vi "VariableGet.vi"(8 "error in (no error)":errorcluster, 10 "VariableName":string, 11 "VariableManager in":refnum<class "VariableManager.lvclass">) -> (0 "error out":errorcluster, 2 "Variable":refnum<class "Variable.lvclass">, 3 "VariableManager out":refnum<class "VariableManager.lvclass">)   [LabVIEW 2013, in "VariableManager.lvclass"]
doc: "Return variable definition of VariableName.\n\nAn error is thrown if a VariableName does not exist."
uses:
  VariableManager.lvclass
  Variable/Variable.lvclass
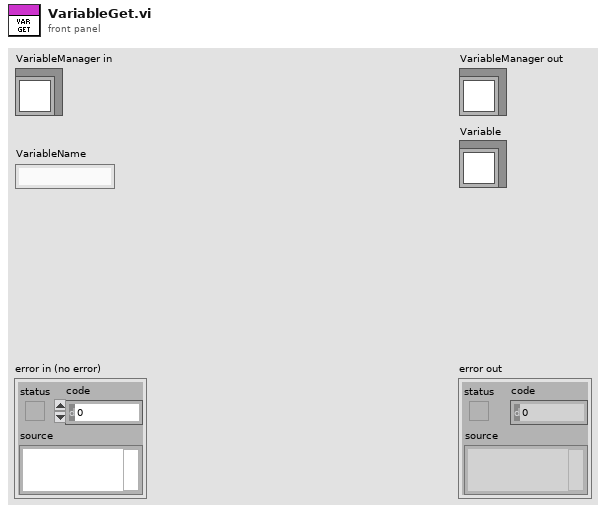
[diagram p1: front panel]
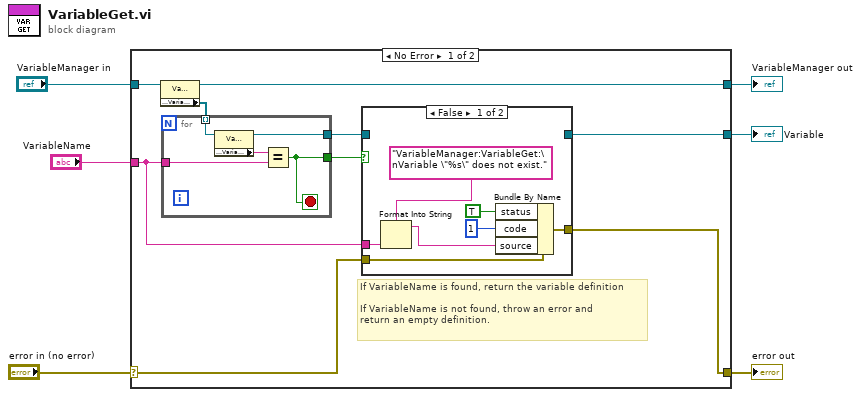
[diagram p0: block diagram]
diagram:
  n1 = case shown="No Error" "error in (no error)" {
    selector: "error in (no error)" -> [w9 w31]
    tunnel: [w8 w31] -> w5
    tunnel: [w14 w30] -> w3
    tunnel: "VariableManager in" -> [w15 w30]
    tunnel: "VariableName" -> [w7 _]
    tunnel: [w11 _] -> w1
    frame No Error {
      # "If VariableName is found, return the variable definition\n\nIf VariableName is not found, throw an error and\nreturn an empty definition."
      n2 = property class="VariableManager.lvclass"(reference=w15) -> (reference out=w14:refnum<class "VariableManager.lvclass">, "Accessors:Variables"=w13:refnum<class "Variable.lvclass">[])  [unwired: 1 in, 1 out]
      n3 = for {
        tunnel: w13 -> [w29] mode=indexing
        tunnel: w7 -> [w27]
        tunnel: [w26] -> w10
        tunnel: [w25] -> w12
        stop <- w26 stop-if-true
        n4 = property class="Variable.lvclass"(reference=w29) -> (reference out=w25:refnum<class "Variable.lvclass">, "Accessors:VariableName"=w28:string)  [unwired: 1 in, 1 out]
        n5 = Equal?(x=w28, y=w27) -> (x = y?=w26:bool)
      }
      n6 = case shown="False" w10 {
        tunnel: w12 -> [_ w23]
        tunnel: [_ w23] -> w11
        tunnel: w9 -> [w22 w24]
        tunnel: w7 -> [w18 _]
        tunnel: [w16 w24] -> w8
        frame False {
          n7 = Format Into String(format string="VariableManager:VariableGet:\nVariable \"%s\" does not exist.", w18) -> (resulting string=w17:string)  [unwired: 2 in, 1 out]
          n8 = Bundle By Name(cluster=w22, "status"=TRUE, "code"=1, "source"=w17) -> (w16:errorcluster)
        }
        frame True {
        }
      }
    }
    frame Error {
    }
  }
  "error out" <- w5
  "VariableManager out" <- w3
  "Variable" <- w1
